vi "counter_channel_consumer.vi"(7 "Sample Group Size":i64, 8 "error in (no error)":errorcluster, 9 "Min. Sampling Window [s]":dbl, 10 "Max. Samping Window [s]":dbl, 11 "Queue in":T1) -> (0 "error out":errorcluster, 2 "Pulse Count":i64, 3 "Pulse Frequency [Hz]":dbl, 4 "Max. Sampling Window Exceeded":bool, 5 "Processed Samples":i32)   [LabVIEW 2025, in "LabJackEKG.lvlib"]
uses:
  LabJackEKG.lvlib
  Typedefs/CounterQueues.ctl
  <vilib>/Analysis/NI_AALPro.lvlib
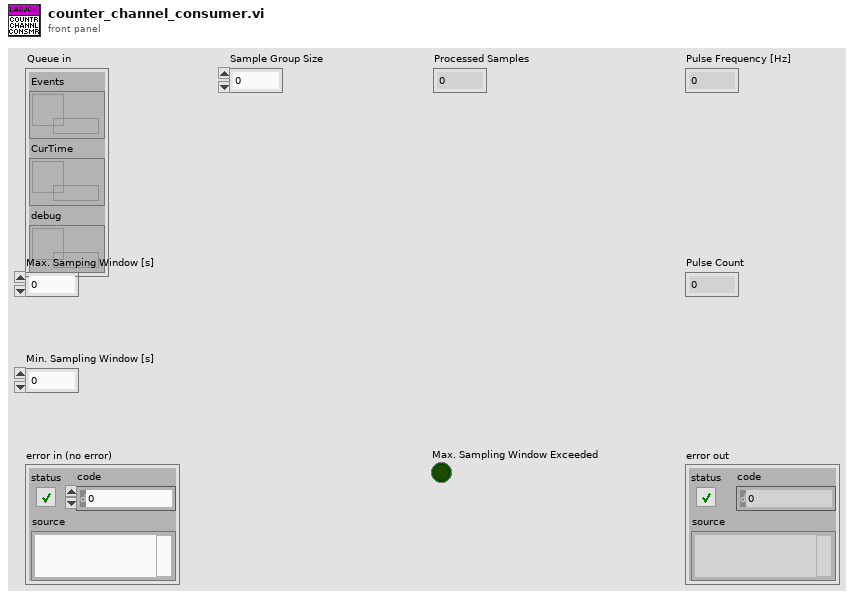
[diagram p1: front panel]
types:
  T1 = typedef "LabJackEKG.lvlib/CounterQueues.ctl" = cluster{"Events":refnum<queue>, "CurTime":refnum<queue>, "debug":refnum<queue>}
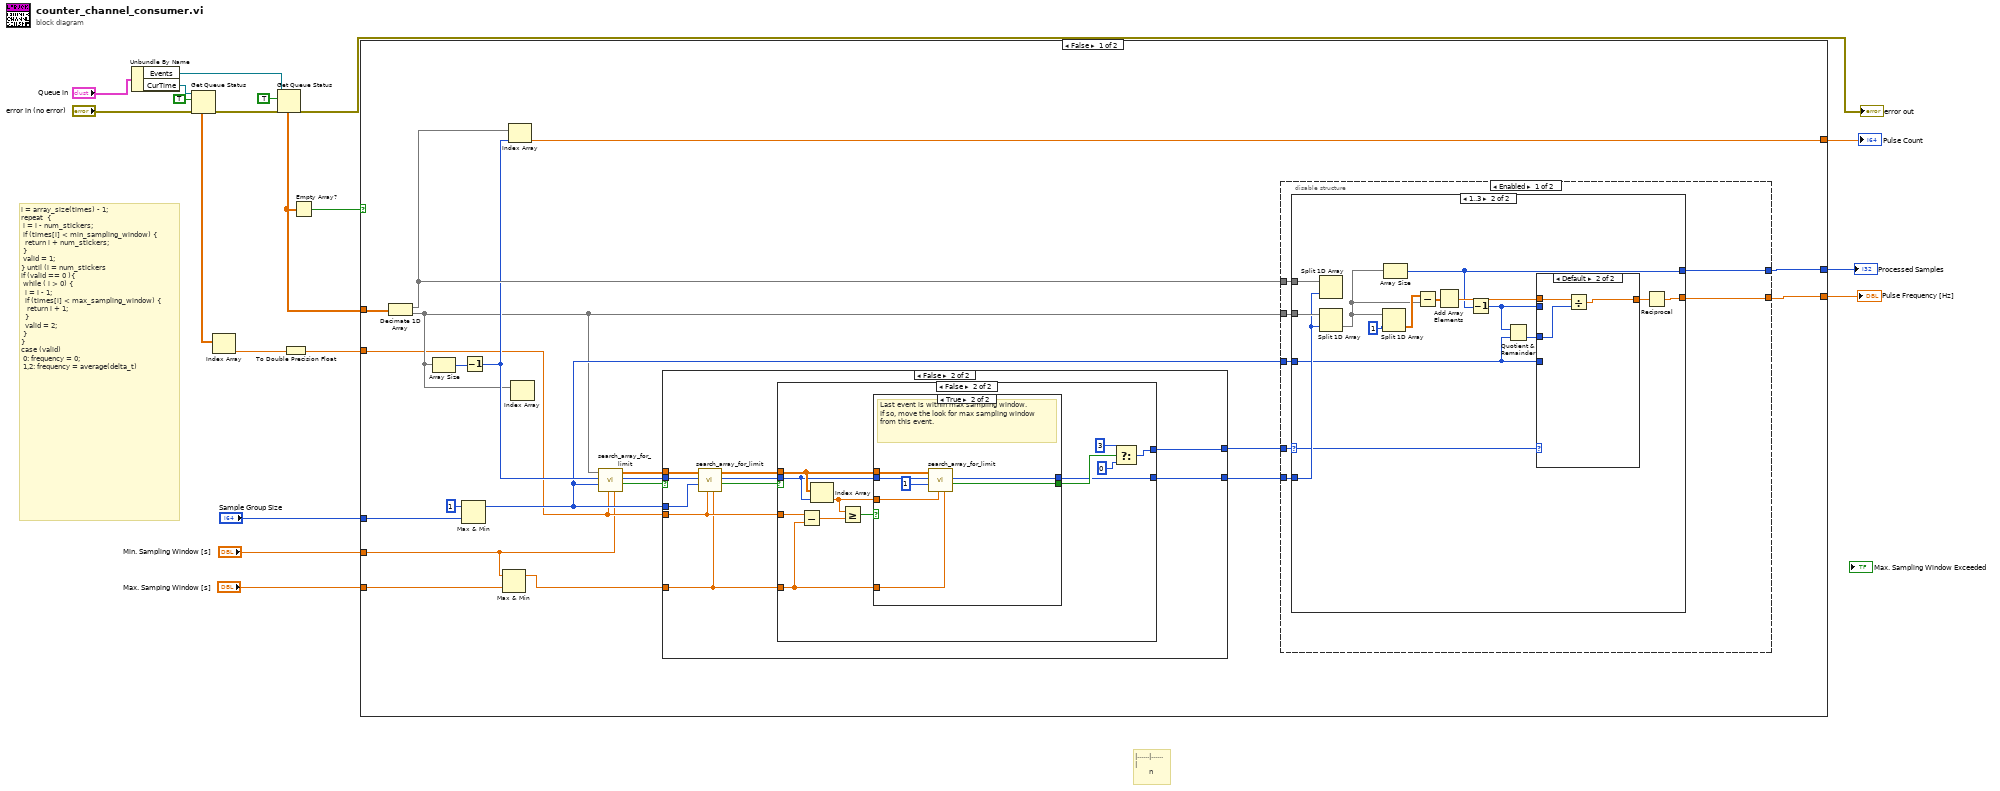
[diagram p0: block diagram]
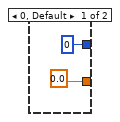
[diagram p2: hidden frame]
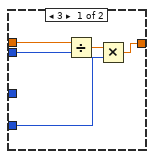
[diagram p3: hidden frame]
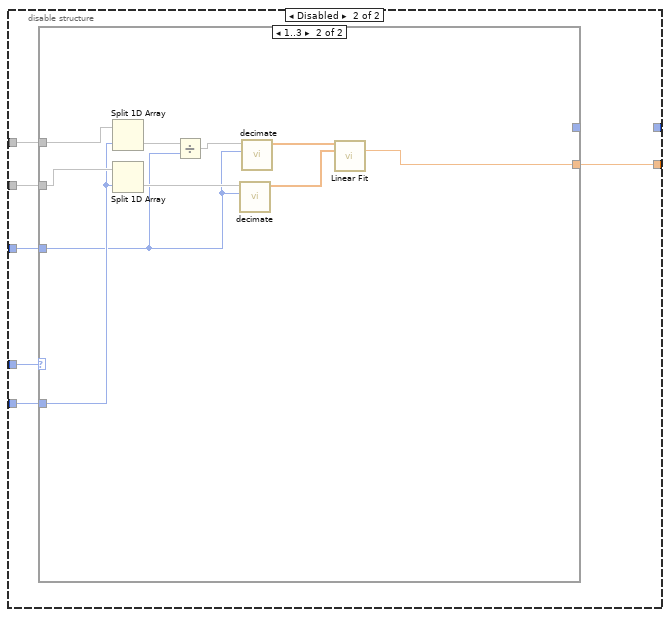
[diagram p4: hidden frame]
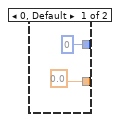
[diagram p5: hidden frame]
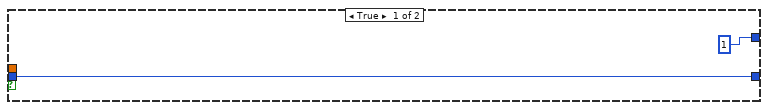
[diagram p6: hidden frame]
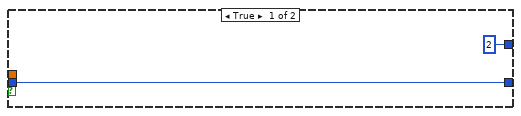
[diagram p7: hidden frame]
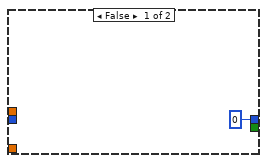
[diagram p8: hidden frame]
diagram:
  # "i = array_size(times) - 1;\nrepeat  {\n\ti = i - num_stickers;\n\tif (times[i] < min_sampling_window) {\n\t\treturn i + num_stickers;\n }\n\tvalid = 1;\n} until (i = num_stickers\nif (valid == 0 ){\n\twhile ( i > 0)\t{\n\t\ti = i - 1;\n\t\tif (times[i] < max_sampling_window)\t{\n\t\t\treturn i + 1;\n\t\t}\n\t\tvalid = 2;\n\t}\n}\ncase (valid)\n\t0: frequency = 0;\n\t1,2: frequency = average(delta_t)"
  # "|......|......|\n       n"
  n1 = Unbundle By Name("Queue in") -> ("Events"=w9:refnum<queue>, "CurTime"=w5:refnum<queue>)
  n2 = Get Queue Status(queue=w5, return elements? (F)=TRUE, error in (no error)="error in (no error)") -> (error out=w6:errorcluster, elements=w3:dbl[])  [unwired: 6 out]
  n3 = Index Array(array=w3) -> (element=w2:dbl)  [unwired: 1 in]
  n4 = Get Queue Status(queue=w9, return elements? (F)=TRUE, error in (no error)=w6) -> (error out=→"error out":errorcluster, elements=w11:dbl[])  [unwired: 6 out]
  n5 = To Double Precision Float(number=w2) -> (double precision float=w1:dbl)
  n6 = Empty Array?(array=w11) -> (empty?=w10:bool)
  n7 = case shown="False" w10 {
    tunnel: "Sample Group Size" -> [w38 _]
    tunnel: [w37 _] -> w16
    tunnel: "Max. Samping Window [s]" -> [w22 _]
    tunnel: "Min. Sampling Window [s]" -> [w21 _]
    tunnel: [w35 _] -> w13
    tunnel: [w23 _] -> w12
    tunnel: w11 -> [w33 _]
    tunnel: w1 -> [w24 _]
    frame False {
      n8 = Decimate 1D Array(w33) -> (w36:dbl[], w25:dbl[])
      n9 = Array Size(array=w25) -> (size(s)=w39:i32)
      n10 = Max & Min(x=i64 1, y=w38) -> (max(x,y)=w31:i64)  [unwired: 1 out]
      n11 = Decrement(x=w39) -> (x-1=w32:i32)
      n12 = Max & Min(x=w21, y=w22) -> (max(x,y)=w20:dbl)  [unwired: 1 out]
      n13 = Index Array(array=w36, index=w32) -> (element=w35:dbl)
      n14 = Index Array(array=w25) -> ()  [unwired: 1 in, 1 out]
      n15 = call "search_array_for_limit.vi"("Window Size"=w21, "Reference Time"=w24, "Step Size"=w31, "Start Index"=w32, "Times"=w25) -> ("Valid"=w30:bool, "End Index"=w29:i32, "Times out"=w28:dbl[])  [unwired: 4 in]
      n16 = case shown="False" w30 {
        tunnel: w31 -> [_ w101]
        tunnel: w29 -> [w90 w100]
        tunnel: w28 -> [_ w99]
        tunnel: [1 ("End Index") w95] -> w27
        tunnel: [w90 w94] -> w26
        tunnel: w24 -> [_ w93]
        tunnel: w20 -> [_ w92]
        frame True {
        }
        frame False {
          n17 = call "search_array_for_limit.vi"("Window Size"=w92, "Reference Time"=w93, "Step Size"=w101, "Start Index"=w100, "Times"=w99) -> ("Valid"=w97:bool, "End Index"=w98:i32, "Times out"=w96:dbl[])  [unwired: 4 in]
          n18 = case shown="False" w97 {
            tunnel: w98 -> [w102 w109]
            tunnel: w96 -> [_ w110]
            tunnel: [2 ("End Index") w113] -> w95
            tunnel: [w102 w111] -> w94
            tunnel: w93 -> [_ w107]
            tunnel: w92 -> [_ w104]
            frame True {
            }
            frame False {
              n19 = Subtract(x=w107, y=w104) -> (x-y=w106:dbl)
              n20 = Index Array(array=w110, index=w109) -> (element=w105:dbl)
              n21 = Greater Or Equal?(x=w105, y=w106) -> (x >= y?=w108:bool)
              n22 = case shown="True" w108 {
                tunnel: [_ w122] -> w115
                tunnel: [0 ("End Index") w121] -> w111
                tunnel: w110 -> [_ w120]
                tunnel: w109 -> [_ w119]
                tunnel: w105 -> [_ w118]
                tunnel: w104 -> [_ w117]
                frame False {
                }
                frame True {
                  # "Last event is within max sampling window. \nIf so, move the look for max sampling window from this event."
                  n23 = call "search_array_for_limit.vi"("Window Size"=w117, "Reference Time"=w118, "Step Size"=1, "Start Index"=w119, "Times"=w120) -> ("Valid"=w122:bool, "End Index"=w121:i32)  [unwired: 4 in, 1 out]
                }
              }
              n24 = Select(t=3 ("End Index"), s=w115, f=0 ("End Index")) -> (s? t:f=w113:i32)
            }
          }
        }
      }
      n25 = disable-structure shown="Enabled" {
        disable-tunnel: [w46 _] -> w37
        disable-tunnel: w36 -> [w45 w77]
        disable-tunnel: w31 -> [w44 w75]
        disable-tunnel: w27 -> [w43 w73]
        disable-tunnel: w26 -> [w42 w72]
        disable-tunnel: w25 -> [w41 w76]
        disable-tunnel: [w40 w74] -> w23
        frame Enabled {
          n26 = case shown="1..3" w43 {
            selector: w43 -> [_ w52]
            tunnel: w41 -> [_ w63]
            tunnel: w45 -> [_ w62]
            tunnel: w42 -> [_ w61]
            tunnel: [0.0 w54] -> w40
            tunnel: [0 w50] -> w46
            tunnel: w44 -> [_ w51]
            frame 0, Default {
            }
            frame 1..3 {
              n27 = Split 1D Array(array=w62, index=w61) -> ()  [unwired: 2 out]
              n28 = Split 1D Array(array=w63, index=w61) -> (second subarray=w53:dbl[])  [unwired: 1 out]
              n29 = Split 1D Array(array=w53, index=1) -> (second subarray=w59:dbl[])  [unwired: 1 out]
              n30 = Array Size(array=w53) -> (size(s)=w50:i32)
              n31 = Subtract(x=w59, y=w53) -> (x-y=w58:dbl[])
              n32 = Add Array Elements(numeric array=w58) -> (sum=w55:dbl)
              n33 = Decrement(x=w50) -> (x-1=w49:i32)
              n34 = Quotient & Remainder(x=w49, y=w51) -> (floor(x/y)=w57:i64)  [unwired: 1 out]
              n35 = case shown="Default" w52 {
                tunnel: w57 -> [_ w71]
                tunnel: [w66 w70] -> w56
                tunnel: w55 -> [w68 w69]
                tunnel: w49 -> [w64 _]
                tunnel: w51 -> [w65 _]
                frame 3 {
                  n36 = Divide(x=w68, y=w64) -> (x/y=w67:dbl)
                  n37 = Multiply(x=w67, y=w65) -> (x*y=w66:dbl)
                }
                frame Default {
                  n38 = Divide(x=w69, y=w71) -> (x/y=w70:dbl)
                }
              }
              n39 = Reciprocal(x=w56) -> (1/x=w54:dbl)
            }
          }
        }
        frame Disabled {
          n40 = case shown="1..3" w73 {
            tunnel: w76 -> [_ w84]
            tunnel: w77 -> [_ w86]
            tunnel: [0.0 w87] -> w74
            tunnel: [0 _] -> _
            tunnel: w75 -> [_ w80]
            tunnel: w72 -> [_ w82]
            frame 0, Default {
            }
            frame 1..3 {
              n41 = Split 1D Array(array=w86, index=w82) -> (second subarray=w85:dbl[])  [unwired: 1 out]
              n42 = Split 1D Array(array=w84, index=w82) -> (second subarray=w83:dbl[])  [unwired: 1 out]
              n43 = Divide(x=w85, y=w80) -> (x/y=w81:dbl[])
              n44 = call "decimate.vi"("Sample Group Size"=w80, "Array in"=w83) -> ("Array out"=w88:dbl[])  [unwired: 9 in]
              n45 = call "decimate.vi"("Sample Group Size"=w80, "Array in"=w81) -> ("Array out"=w89:dbl[])  [unwired: 9 in]
              n46 = call <vilib>:"Linear Fit.vi"("Y"=w89, "X"=w88) -> ("slope"=w87:dbl)  [unwired: 9 in, 4 out]
            }
          }
        }
      }
    }
    frame True {
    }
  }
  "Pulse Frequency [Hz]" <- w12
  "Processed Samples" <- w16
  "Pulse Count" <- w13
